vi "注册设备.vi"(6 "待注册设备MAC":string, 7 "企业数据库":string, 8 "error in (no error)":errorcluster, 11 "数据库引用.i":T1) -> (0 "error out":errorcluster, 3 "数据库引用.o":T1)   [LabVIEW 2013, in "数据库操作.lvclass"]
uses:
  <vilib>/addons/database/Connection.llb/Conn ObjectReference.ctl
  <vilib>/addons/database/Connection.llb/Conn Execute.vi
  <vilib>/addons/database/NI_Database_API.lvlib
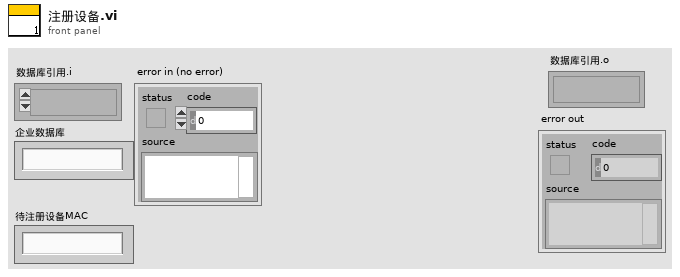
[diagram p1: front panel]
types:
  T1 = typedef "NI_Database_API.lvlib/Conn ObjectReference.ctl" = refnum<k1>
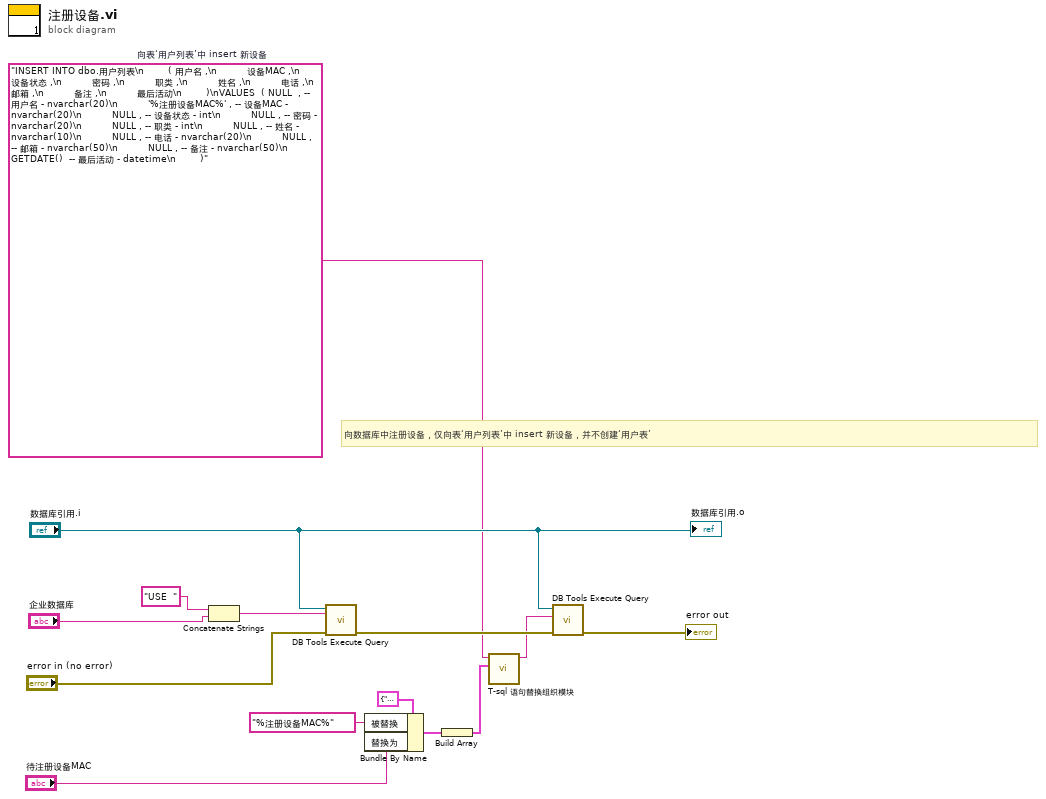
[diagram p0: block diagram]
diagram:
  w8 = "INSERT INTO dbo.用户列表\n        ( 用户名 ,\n          设备MAC ,\n          设备状态 ,\n          密码 ,\n          职类 ,\n          姓名 ,\n          电话 ,\n          邮箱 ,\n          备注 ,\n          最后活动\n        )\nVALUES  ( NULL  , -- 用户名 - nvarchar(20)\n          '%注册设备MAC%' , -- 设备MAC - nvarchar(20)\n          NULL , -- 设备状态 - int\n          NULL , -- 密码 - nvarchar(20)\n          NULL , -- 职类 - int\n          NULL , -- 姓名 - nvarchar(10)\n          NULL , -- 电话 - nvarchar(20)\n          NULL , -- 邮箱 - nvarchar(50)\n          NULL , -- 备注 - nvarchar(50)\n          GETDATE()  -- 最后活动 - datetime\n        )"  # 向表‘用户列表’中 insert 新设备
  # "向数据库中注册设备，仅向表‘用户列表’中 insert 新设备，并不创建‘用户表’"
  n1 = Concatenate Strings("USE  " ("字符串"), "企业数据库") -> (w11:string)
  n2 = call-poly <vilib>:"DB Tools Execute Query.vi"("error in (no error)"="error in (no error)", "SQL query"=w11, "connection reference"="数据库引用.i") -> ("error out"=w9:errorcluster)  [unwired: 5 in, 1 out]
  n3 = Bundle By Name(cluster=cluster{"被替换":string, "替换为":string} {"被替换"="", "替换为"=""} ("替换单元"), "被替换"="%注册设备MAC%", "替换为"="待注册设备MAC") -> (w4:cluster{"被替换":string, "替换为":string})
  n4 = Build Array(w4) -> (w3:cluster{"被替换":string, "替换为":string}[])
  n5 = call "T-sql 语句替换组织模块.vi"("替换项"=w3, "T-sql 模板"=w8) -> ("T-sql"=w2:string)  [unwired: 8 in, 1 out]
  n6 = call-poly <vilib>:"DB Tools Execute Query.vi"("error in (no error)"=w9, "SQL query"=w2, "connection reference"="数据库引用.i") -> ("error out"=→"error out":errorcluster)  [unwired: 5 in, 1 out]
  "数据库引用.o" <- "数据库引用.i"
